vi "CloseAll.vi"(8 "error in (no error)":errorcluster) -> (0 "error out":errorcluster)   [LabVIEW 2024, in "LogSingleton.lvlib"]
uses:
  LogSingleton.lvlib
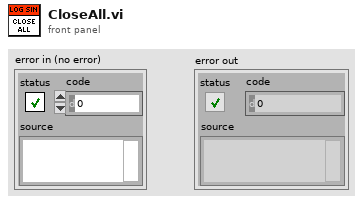
[diagram p1: front panel]
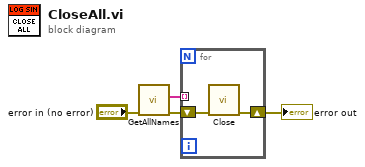
[diagram p0: block diagram]
diagram:
  n1 = call "GetAllNames.vi"("error in (no error)"="error in (no error)") -> ("error out"=w4:errorcluster, "Keys"=w3:string[])  [unwired: 9 in]
  n2 = for {
    shift-right: [w5] -> w2
    shift-left: w4 -> [w6]
    tunnel: w3 -> [_] mode=indexing
    n3 = call "Close.vi"("error in (no error)"=w6) -> ("error out"=w5:errorcluster)  [unwired: 10 in]
  }
  "error out" <- w2
